vi "Tarea 2.6 VI.vi"() -> ()   [LabVIEW 2013]
uses:
  <vilib>/Instr/_visa.llb/VISA Configure Serial Port (Instr).vi
panel:
  out "Caso":dbl
  in  "Letter":string
  out "LINE OUT":string
  in  "SW":bool[](array[boolean])
  in  "Start Com":bool
  in  "Stop Button":bool
  # "COMANDOS RESERVADOS\nS para Iniciar\nE para terminar."
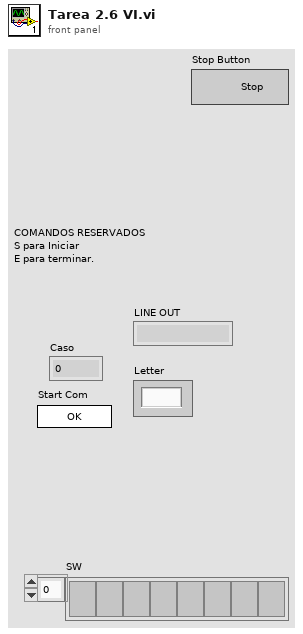
[diagram p1: front panel]
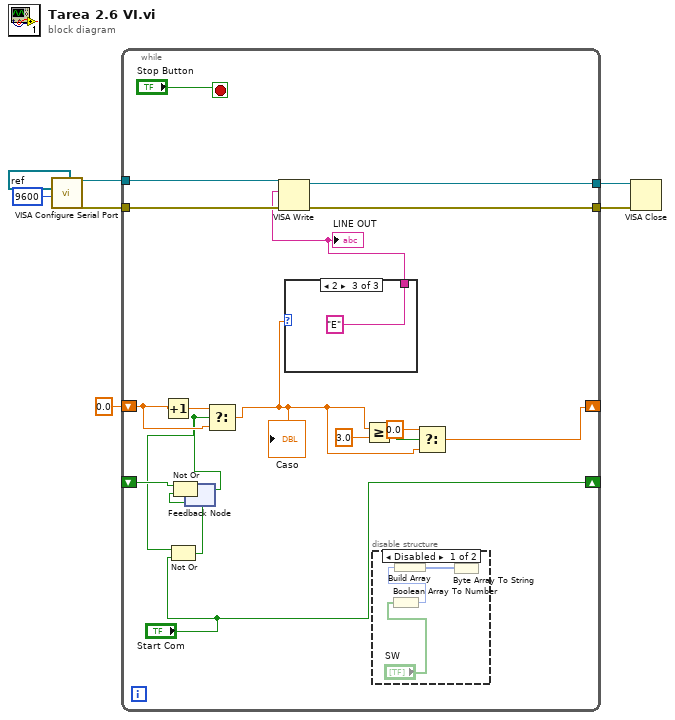
[diagram p0: block diagram]
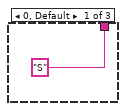
[diagram p2: hidden frame]
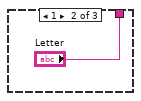
[diagram p3: hidden frame]
diagram:
  n1 = call-poly "VISA Configure Serial Port"("VISA resource name"=refnum<visa-resource-name> "COM6", "baud rate (9600)"=u32 9600) -> ("VISA resource name out"=w7:refnum<visa-resource-name>, "error out"=w6:errorcluster)  [unwired: 12 in]
  n2 = while {
    tunnel: w7 -> [w24]
    tunnel: w6 -> [w23]
    tunnel: [w22] -> w3
    tunnel: [w21] -> w2
    shift-right: ["Start Com"] -> _
    shift-left: _ -> [w20]
    shift-right: [w8] -> _
    shift-left: 0.0 -> [w18]
    stop <- "Stop Button" stop-if-true
    n3 = Increment(x=w18) -> (x+1=w19:dbl)
    n4 = feedback #1() -> (w15:bool)  [unwired: 1 in]
    n5 = Not Or(1:"Start Com", 2:w15) -> (0:w17:bool)
    n6 = Not Or(1:w17, 2:w20) -> (0:w16:bool)
    n7 = feedback-in #1(w16) -> ()
    n8 = Select(t=w19, s=w15, f=w18) -> (s? t:f=w9:dbl)
    "Caso" <- w9
    n9 = case shown="2" w9 {
      tunnel: ["S" "Letter" "E"] -> w13
      frame 0, Default {
      }
      frame 1 {
      }
      frame 2 {
      }
    }
    "LINE OUT" <- w13
    n10 = VISA Write(VISA resource name=w24, write buffer=w13, error in (no error)=w23) -> (VISA resource name out=w22:refnum<visa-resource-name>, error out=w21:errorcluster)  [unwired: 1 out]
    n11 = Greater Or Equal?(x=w9, y=3.0) -> (x >= y?=w11:bool)
    n12 = disable-structure shown="Disabled" {
      frame Disabled {
        n13 = Boolean Array To Number(Boolean array="SW") -> (number=w30:u32)
        n14 = Build Array(w30) -> (w31:u32[])
        n15 = Byte Array To String(unsigned byte array=w31) -> ()  [unwired: 1 out]
      }
      frame Enabled {
      }
    }
    n16 = Select(t=0.0, s=w11, f=w9) -> (s? t:f=w8:dbl)
  }
  n17 = VISA Close(VISA resource name=w3, error in (no error)=w2) -> ()  [unwired: 1 out]
